vi "IR Emitter Test.vi"(5 "Test Configuration":T1, 8 "error in (no error)":errorcluster, 11 "Session Handle in":T8) -> (0 "error out":errorcluster, 1 "Failure Reason":string, 2 "Passed?":bool, 3 "Session Handle out":T8)   [LabVIEW 2015, in "PAS.lvclass"]
uses:
  PAS.lvclass
  Typedefs/Session Handle.ctl
  Tests/Controls/Test Configuration.ctl
  Tests/Controls/Vacuum Test.ctl
  Tests/Controls/Test Timing.ctl
  Tests/Controls/Vaccum Thresholds.ctl
  Tests/Controls/Helium Test.ctl
  Tests/Controls/Helium Thresholds.ctl
  Tests/Controls/Functional Test.ctl
  Typedefs/Emitter Power.ctl
  Typedefs/Valves.ctl
panel:
  out "Passed?":bool
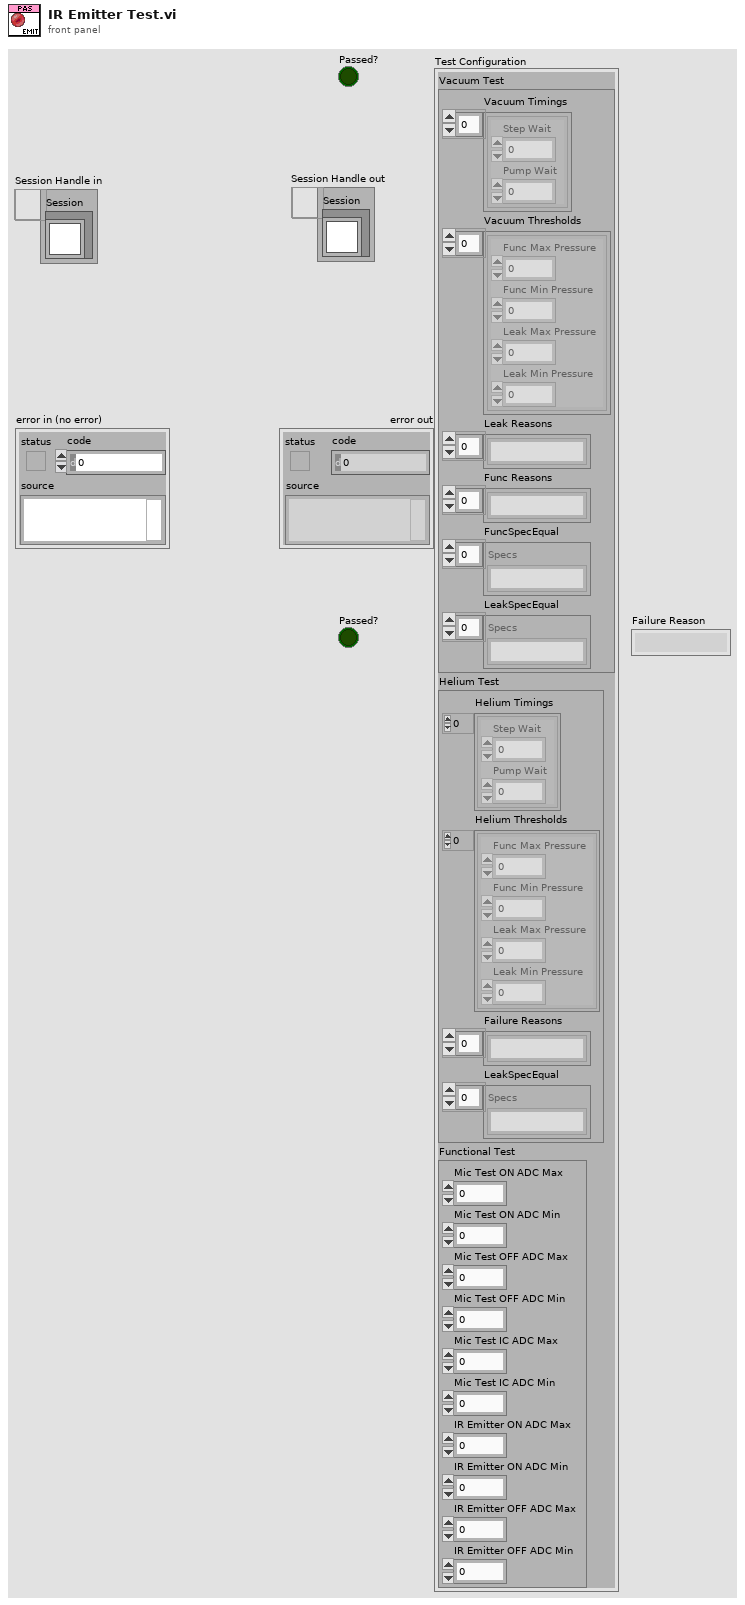
[diagram p1: front panel]
types:
  T1 = typedef "Test Configuration.ctl" = cluster{"Vacuum Test":T2, "Helium Test":T5, "Functional Test":T7}
  T2 = typedef "Vacuum Test.ctl" = cluster{"Vacuum Timings":T3[], "Vacuum Thresholds":T4[], "Leak Reasons":string[], "Func Reasons":string[], "FuncSpecEqual":string[], "LeakSpecEqual":string[]}
  T3 = typedef "Test Timing.ctl" = cluster{"Step Wait":dbl, "Pump Wait":dbl}
  T4 = typedef "Vaccum Thresholds.ctl" = cluster{"Func Max Pressure":dbl, "Func Min Pressure":dbl, "Leak Max Pressure":dbl, "Leak Min Pressure":dbl}
  T5 = typedef "Helium Test.ctl" = cluster{"Helium Timings":T3[], "Helium Thresholds":T6[], "Failure Reasons":string[], "LeakSpecEqual":string[]}
  T6 = typedef "Helium Thresholds.ctl" = cluster{"Func Max Pressure":dbl, "Func Min Pressure":dbl, "Leak Max Pressure":dbl, "Leak Min Pressure":dbl}
  T7 = typedef "Functional Test.ctl" = cluster{"Mic Test ON ADC Max":dbl, "Mic Test ON ADC Min":dbl, "Mic Test OFF ADC Max":dbl, "Mic Test OFF ADC Min":dbl, "Mic Test IC ADC Max":dbl, "Mic Test IC ADC Min":dbl, "IR Emitter ON ADC Max":dbl, "IR Emitter ON ADC Min":dbl, "IR Emitter OFF ADC Max":dbl, "IR Emitter OFF ADC Min":dbl}
  T8 = typedef "PAS.lvclass/Session Handle.ctl" = refnum<data-value>
  T9 = typedef "PAS.lvclass/Valves.ctl" = u16
  T10 = typedef "PAS.lvclass/Emitter Power.ctl" = u16
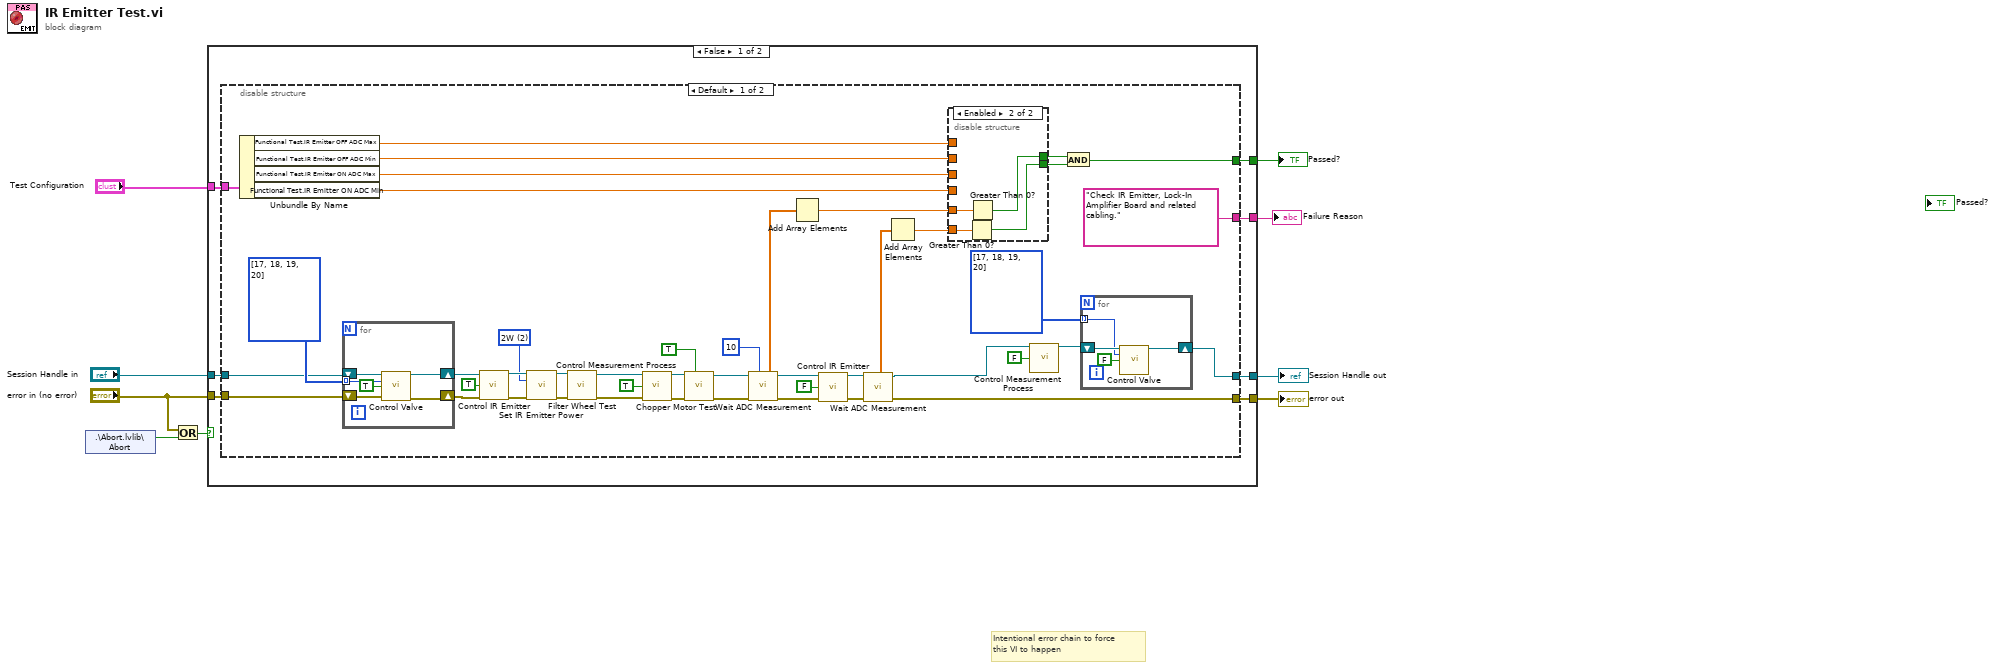
[diagram p0: block diagram]
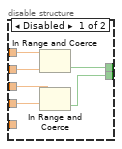
[diagram p2: hidden frame]
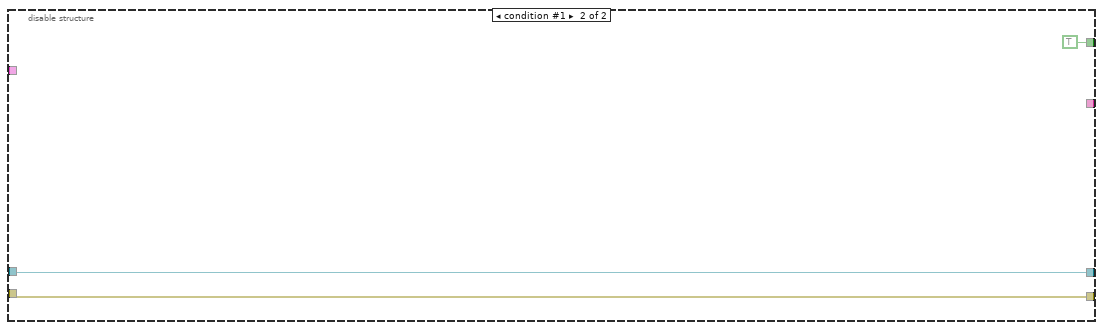
[diagram p3: hidden frame]
diagram:
  # "Intentional error chain to force\nthis VI to happen"
  n1 = shared-variable ".\\Abort.lvlib\\Abort"() -> (w3:bool)  [unwired: 1 in, 1 out]
  n2 = Or(x="error in (no error)", y=w3) -> (x .or. y?=w4:bool)
  n3 = case shown="False" w4 {
    tunnel: "error in (no error)" -> [w16 w84]
    tunnel: [w15 w85] -> w9
    tunnel: "Session Handle in" -> [w14 w85]
    tunnel: "Test Configuration" -> [w13 _]
    tunnel: [w12 w84] -> w6
    tunnel: [w11 _] -> w5
    tunnel: [w10 _] -> w1
    frame False {
      n4 = disable-structure shown="Default" {
        disable-tunnel: w16 -> [w60 w83]
        disable-tunnel: [w50 w82] -> w15
        disable-tunnel: w14 -> [w49 w82]
        disable-tunnel: w13 -> [w48 _]
        disable-tunnel: [w21 w83] -> w12
        disable-tunnel: [w31 TRUE] -> w11
        disable-tunnel: ["Check IR Emitter, Lock-In Amplifier Board and related cabling." ("t") _] -> w10
        frame condition #0 (active) {
          w38 = T9[] [17, 18, 19, 20] items=["PV1"=17, "PV2"=18, "PV3"=19, "PV4"=20]
          w53 = T10 2 items=["2W"=2, "3W"=3, "4W"=4, "5W"=5] ("Emitter Power")
          w59 = T9[] [17, 18, 19, 20] items=["PV1"=17, "PV2"=18, "PV3"=19, "PV4"=20]
          n5 = Unbundle By Name(w48) -> ("Functional Test.IR Emitter OFF ADC Max"=w35:dbl, "Functional Test.IR Emitter OFF ADC Min"=w34:dbl, "Functional Test.IR Emitter ON ADC Max"=w37:dbl, "Functional Test.IR Emitter ON ADC Min"=w36:dbl)
          n6 = for {
            shift-right: [w76] -> w58
            shift-left: w49 -> [w80]
            shift-right: [w77] -> w57
            shift-left: w60 -> [w78]
            tunnel: w59 -> [w79] mode=indexing
            n7 = call "Control Valve.vi"("Session Handle in"=w80, "Valves"=w79, "Energize?"=TRUE, "error in (no error)"=w78) -> ("Session Handle out"=w76:T8, "error out"=w77:errorcluster)  [unwired: 8 in, 2 out]
          }
          n8 = call "Control IR Emitter.vi"("Session Handle in"=w58, "Start?"=TRUE, "error in (no error)"=w57) -> ("Session Handle out"=w55:T8, "error out"=w54:errorcluster)  [unwired: 9 in, 2 out]
          n9 = call "Set IR Emitter Power.vi"("Session Handle in"=w55, "Emitter Power"=w53, "error in (no error)"=w54) -> ("Session Handle out"=w47:T8, "error out"=w46:errorcluster)  [unwired: 10 in, 1 out]
          n10 = call "Filter Wheel Test.vi"("error in (no error)"=w46, "Session Handle in"=w47) -> ("error out"=w41:errorcluster, "Session Handle out"=w42:T8)  [unwired: 7 in, 1 out]
          n11 = call "Control Measurement Process.vi"("Session Handle in"=w42, "Start?"=TRUE, "error in (no error)"=w41) -> ("Session Handle out"=w44:T8, "error out"=w43:errorcluster)  [unwired: 9 in, 2 out]
          n12 = call "Chopper Motor Test.vi"("Measurement Started?"=TRUE, "error in (no error)"=w43, "Session Handle in"=w44) -> ("error out"=w28:errorcluster, "Session Handle out"=w29:T8)  [unwired: 6 in, 1 out]
          n13 = call "Wait ADC Measurement.vi"("Wait (s)"=10, "error in (no error)"=w28, "Session Handle in"=w29) -> ("error out"=w27:errorcluster, "Array"=w24:dbl[], "Session Handle out"=w26:T8)  [unwired: 5 in, 1 out]
          n14 = Add Array Elements(numeric array=w24) -> (sum=w18:dbl)
          n15 = call "Control IR Emitter.vi"("Session Handle in"=w26, "Start?"=FALSE, "error in (no error)"=w27) -> ("Session Handle out"=w23:T8, "error out"=w22:errorcluster)  [unwired: 9 in, 2 out]
          n16 = call "Wait ADC Measurement.vi"("error in (no error)"=w22, "Session Handle in"=w23) -> ("error out"=w21:errorcluster, "Array"=w19:dbl[], "Session Handle out"=w20:T8)  [unwired: 6 in, 1 out]
          n17 = Add Array Elements(numeric array=w19) -> (sum=w17:dbl)
          n18 = disable-structure shown="Enabled" {
            disable-tunnel: w37 -> [w66 _]
            disable-tunnel: w36 -> [w65 _]
            disable-tunnel: w35 -> [w64 _]
            disable-tunnel: w34 -> [w63 _]
            disable-tunnel: [w62 w68] -> w33
            disable-tunnel: [w61 w67] -> w32
            disable-tunnel: w18 -> [_ w70]
            disable-tunnel: w17 -> [_ w69]
            frame Disabled {
              n19 = In Range and Coerce(upper limit=w64, lower limit=w63) -> (In Range?=w62:bool)  [unwired: 1 in, 1 out]
              n20 = In Range and Coerce(upper limit=w66, lower limit=w65) -> (In Range?=w61:bool)  [unwired: 1 in, 1 out]
            }
            frame Enabled {
              n21 = Greater Than 0?(x=w69) -> (x > 0?=w67:bool)
              n22 = Greater Than 0?(x=w70) -> (x > 0?=w68:bool)
            }
          }
          n23 = call "Control Measurement Process.vi"("Session Handle in"=w20, "Start?"=FALSE) -> ("Session Handle out"=w51:T8)  [unwired: 10 in, 3 out]
          n24 = And(x=w33, y=w32) -> (x .and. y?=w31:bool)
          n25 = for {
            shift-right: [w73] -> w50
            shift-left: w51 -> [w74]
            tunnel: w38 -> [w71] mode=indexing
            n26 = call "Control Valve.vi"("Session Handle in"=w74, "Valves"=w71, "Energize?"=FALSE) -> ("Session Handle out"=w73:T8)  [unwired: 9 in, 3 out]
          }
        }
        frame condition #1 {
        }
      }
    }
    frame True {
    }
  }
  "error out" <- w6
  "Session Handle out" <- w9
  "Passed?" <- w5
  "Failure Reason" <- w1
